vi "Menu - Set Checked State.vi"(6 "State":enum16{"Unchecked", "Checked"}(ring), 8 "error in (no error)":errorcluster, 10 "item tag":string, 11 "menu reference":refnum<k9>) -> (0 "error out":errorcluster)   [LabVIEW 2015]
doc: "Sets the Checked? state of the desired menu item."
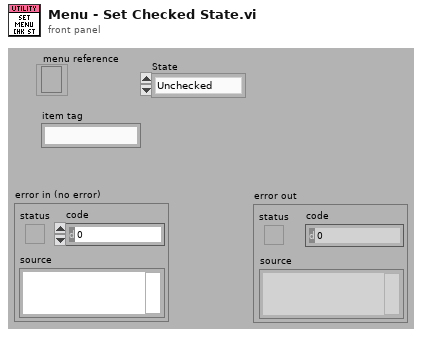
[diagram p1: front panel]
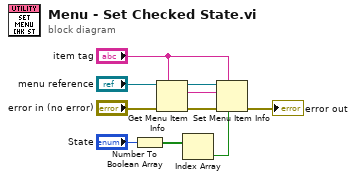
[diagram p0: block diagram]
diagram:
  n1 = Number To Boolean Array(number="State") -> (Boolean array=w2:bool[])
  n2 = Get Menu Item Info(7:"item tag", 8:"error in (no error)", 11:"menu reference") -> (0:w5:errorcluster, 2:w9:string, 3:w10:refnum<k9>)  [unwired: 4 out]
  n3 = Index Array(array=w2) -> (element=w1:bool)  [unwired: 1 in]
  n4 = Set Menu Item Info(6:w1, 7:"item tag", 8:w5, 10:w9, 11:w10) -> (0:→"error out":errorcluster)  [unwired: 3 out]
